vi "Explain DVR Error.vi"(8 "error in (no error)":errorcluster) -> (0 "error out":errorcluster)   [LabVIEW 2017, in "Configuration.lvlib" / "ConfigurationReference.lvclass"]
uses:
  ConfigurationReference.lvclass
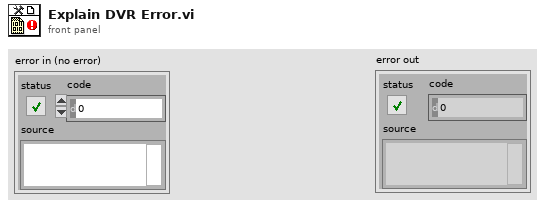
[diagram p1: front panel]
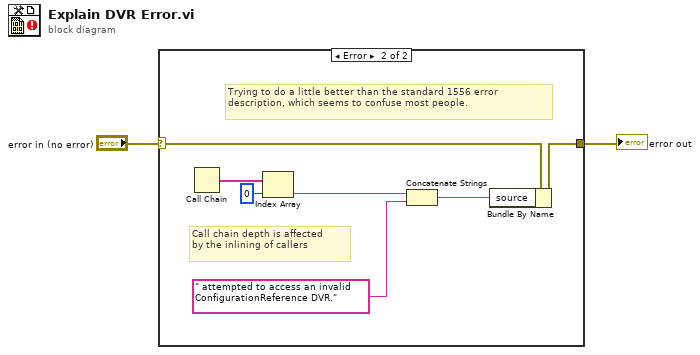
[diagram p0: block diagram]
diagram:
  n1 = case shown="Error" "error in (no error)" {
    selector: "error in (no error)" -> [w3 w10]
    tunnel: [w3 w9] -> w1
    frame No Error {
    }
    frame Error {
      # "Call chain depth is affected\nby the inlining of callers"
      # "Trying to do a little better than the standard 1556 error\ndescription, which seems to confuse most people."
      n2 = Call Chain() -> (call chain=w8:string[])
      n3 = Index Array(array=w8, index=0) -> (element=w6:string)
      n4 = Concatenate Strings(w6, " attempted to access an invalid ConfigurationReference DVR." ("source")) -> (w4:string)
      n5 = Bundle By Name(cluster=w10, "source"=w4) -> (w9:errorcluster)
    }
  }
  "error out" <- w1
